vi "ADAM_scan_table.vi"() -> ()   [LabVIEW 2013]
uses:
  Anemometry/Anemometry Sub Vis/Controls/Serveds.ctl
  ADAM Client/Sub VIs/ADAM Controls/Module_type_ADAM.ctl
  ADAM Client/Sub VIs/ADAM Controls/Traverse_Level_State.ctl
  Anemometry/Anemometry Sub Vis/Controls/Post_Process.ctl
  ADAM Client/Sub VIs/ADAM Controls/Channel_State.ctl
  ADAM Client/Sub VIs/ADAM Controls/Ch_description_ADAM.ctl
  ADAM Client/Sub VIs/ADAM Controls/Function_ADAM.ctl
  ADAM Client/Sub VIs/ADAM Controls/Calib_type_ADAM.ctl
  ADAM Client/Sub VIs/ADAM Controls/Address.ctl
  ADAM_Global.vi
  Sub VI's/Channel_Description_Global.vi
  Anemometry/Anemometry Sub Vis/Globals/Meas_global.vi
  Sub VI's/Logged_Data_real_Global.vi
  Anemometry/Anemometry Sub Vis/Globals/Preference_global.vi
  Anemometry/Anemometry Sub Vis/Globals/Gas_management_global.vi
  Anemometry/Anemometry Sub Vis/Globals/Constants_global.vi
panel:
  in  "Reconfigure Gills":bool
  in  "Full Res Pathname":path
  in  "Log full Res Data":bool
  out "Duty No":u16 format="%.0b"
  in  "Save Current setup":bool=TRUE
  in  "Load setup from file":bool
  out "ADAM scan comments":string
  out "History length":i32=250
  in  "stop":bool
  out "Results":dbl[](array[numeric]) format="%.3f"
  out "Titles":string[](array[string])
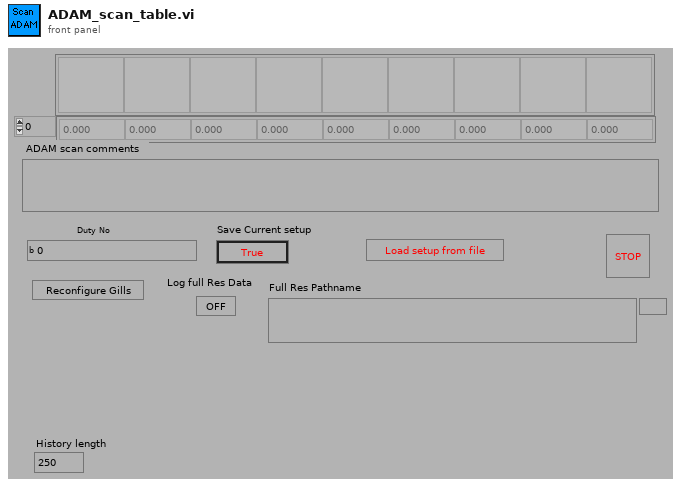
[diagram p1: front panel]
types:
  T1 = enum16{"Load ADAM setup from excel file", "Save ADAM setup to excel file"}
  T2 = typedef "Serveds.ctl" = enum16{"Read Global", "Load Global From File"}
  T3 = typedef "Module_type_ADAM.ctl" = string
  T4 = typedef "Traverse_Level_State.ctl" = enum16{"Running", "Complete"}
  T5 = typedef "Post_Process.ctl" = enum16{"Take New Data", "Post Process Raw Data File"}
  T6 = typedef "Channel_State.ctl" = enum16{"On", "Off", "Always On", "Always Off"}
  T7 = enum16{"Append to Global", "Read Global then Clear"}
  T8 = typedef "Ch_description_ADAM.ctl" = cluster{"Ch Name":string, "Type":T3, "Function":T9, "Ch State":T6, "Calibration type":T10, "A":dbl, "B":dbl, "C":dbl, "D":dbl, "Comments":string, "Address":T11, "String":string, "Duty":u16}
  T9 = typedef "Function_ADAM.ctl" = enum16{"Analogue Input", "Digital Input", "Event counter", "Event rate", "Analogue Output", "Digital Output", "Relay Output"}
  T10 = typedef "Calib_type_ADAM.ctl" = enum16{"Raw", "Bx + A", "Cx^2 + Bx + A", "Dx^3 + Cx^2 + Bx + A", "In Band", "Hi-Tec Q", "Hi-Tec M_dot", "Text"}
  T11 = typedef "Address.ctl" = cluster{"Main":i32, "Ch.":i32, "Sub":i32, "Port Name":string}
  T12 = typedef "Client_State_Cluster.ctl" = cluster{"Client Name":string, "Traverse level State":T4, "People to Email":string[], "Next Contact Time":dbl}
  T13 = typedef "ADAM_Comparitor.ctl" = cluster{"Ch to Monitor":string, "Channels to Kill":string, "Warn if Above":dbl, "Warn if Below":dbl, "Kill if Above":dbl, "Kill if Below":dbl, "Hysteresis Margin":dbl, "Averaging TIme (s)":dbl, "Warn Status":bool, "Kill Status":bool, "Extra Email addresses":string}
  T14 = typedef "Update_scan_value.ctl" = cluster{"Channel Name":string, "New Value":dbl}
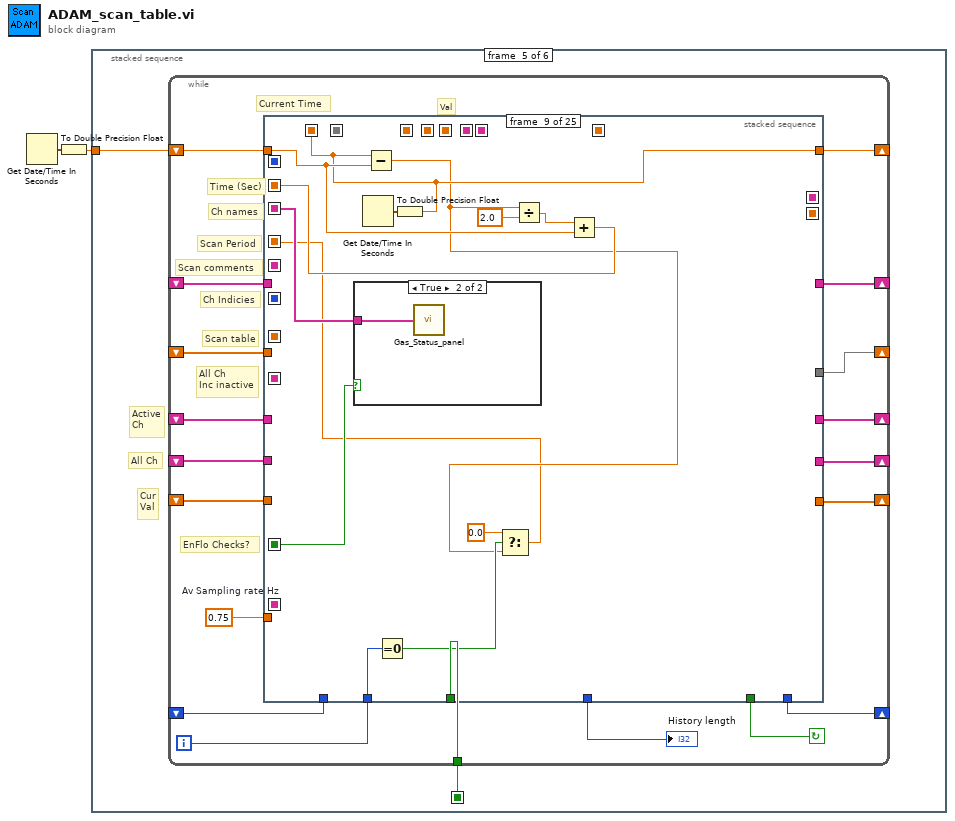
[diagram p0: block diagram]
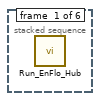
[diagram p2: hidden frame]
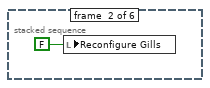
[diagram p3: hidden frame]
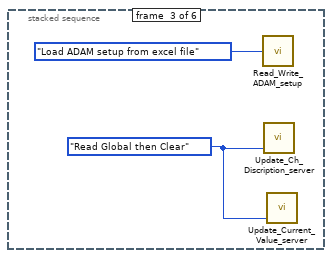
[diagram p4: hidden frame]
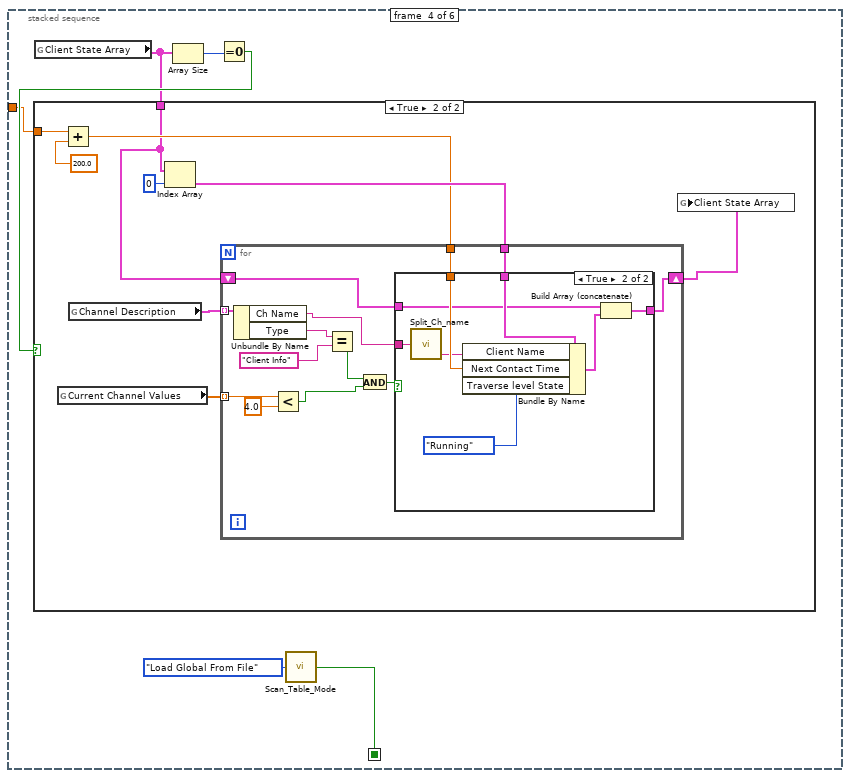
[diagram p5: hidden frame]
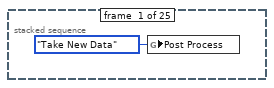
[diagram p8: hidden frame]
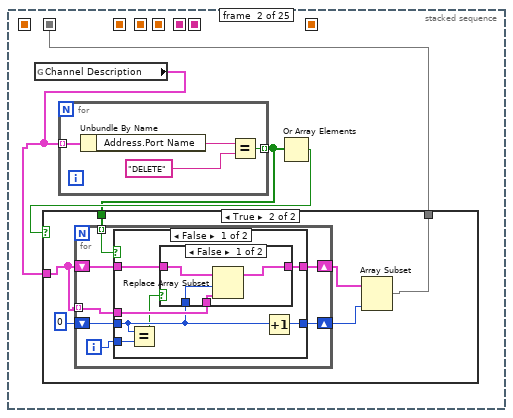
[diagram p9: hidden frame]
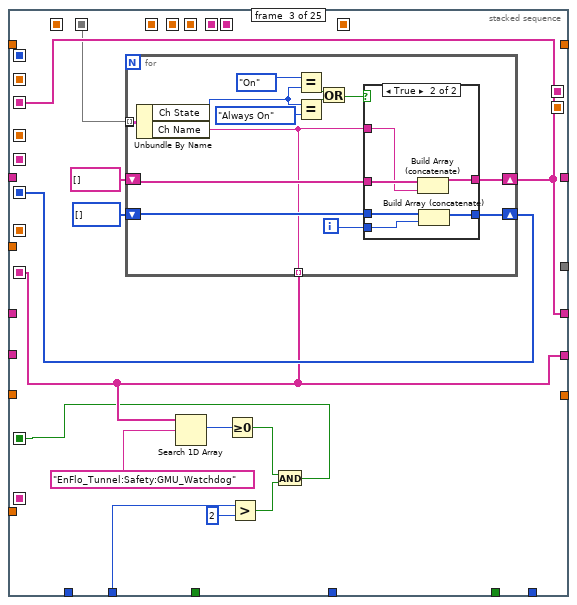
[diagram p13: hidden frame]
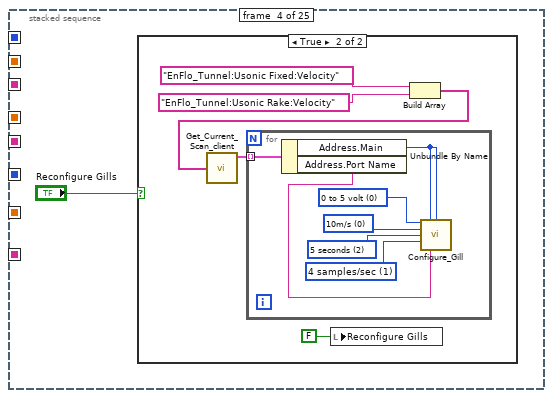
[diagram p15: hidden frame]
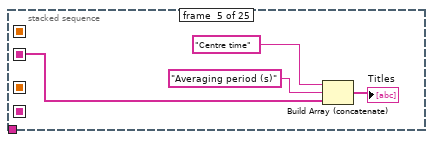
[diagram p17: hidden frame]
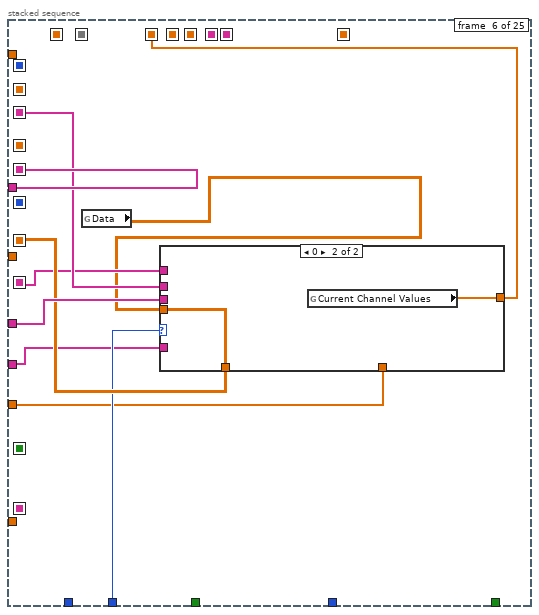
[diagram p18: hidden frame]
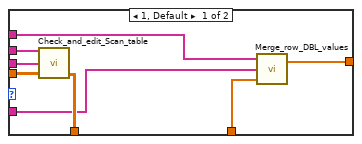
[diagram p19: hidden frame]
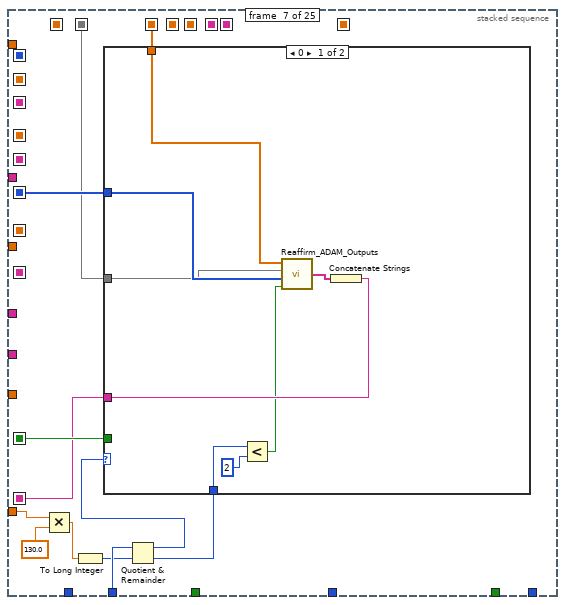
[diagram p20: hidden frame]
diagram:
  n1 = Get Date/Time In Seconds() -> (seconds since 1Jan1904=w2:timestamp)
  n2 = To Double Precision Float(number=w2) -> (double precision float=w1:dbl)
  n3 = stacked-sequence {
    seq-local: [_ _ _ w11 _ _] -> [_ _ _ _ w44 _]
    tunnel: w1 -> [_ _ _ w6 w43 _]
    frame #0 {
      n4 = call "Run_EnFlo_Hub.vi"() -> ()  [unwired: 8 out]
    }
    frame #1 {
      n5 = local write "Reconfigure Gills"(FALSE ("Reconfigure Gills")) -> ()
    }
    frame #2 {
      w4 = T7."Read Global then Clear" ("Mode")
      n6 = call "Read_Write_ADAM_setup.vi"("Mode"=T1."Load ADAM setup from excel file") -> ()  [unwired: 4 out]
      n7 = call "Update_Ch_Discription_server.vi"("Mode"=w4) -> ()  [unwired: 2 in, 1 out]
      n8 = call "Update_Current_Value_server.vi"("Mode"=w4) -> ()  [unwired: 2 in, 1 out]
    }
    frame #3 {
      n9 = global read "ADAM_Global.vi" "Client State Array"() -> (w7:T12[])
      n10 = Array Size(array=w7) -> (size(s)=w9:i32)
      n11 = Equal To 0?(x=w9) -> (x = 0?=w8:bool)
      n12 = case shown="True" w8 {
        tunnel: w7 -> [_ w13]
        tunnel: w6 -> [_ w16]
        frame False {
        }
        frame True {
          n13 = global read "ADAM_Global.vi" "Current Channel Values"() -> (w20:dbl[])
          n14 = Add(x=w16, y=200.0) -> (x+y=w14:dbl)
          n15 = global read "Channel_Description_Global.vi" "Channel Description"() -> (w19:T8[])
          n16 = Index Array(array=w13, index=0) -> (element=w17:T12)
          n17 = for {
            tunnel: w19 -> [w33] mode=indexing
            tunnel: w20 -> [w25] mode=indexing
            tunnel: w17 -> [w26]
            tunnel: w14 -> [w24]
            shift-right: [w23] -> w12
            shift-left: w13 -> [w22]
            n18 = Unbundle By Name(w33) -> ("Ch Name"=w21:string, "Type"=w30:T3)
            n19 = Less?(x=w25, y=4.0) -> (x < y?=w28:bool)
            n20 = Equal?(x=w30, y=T3 "Client Info" ("Type")) -> (x = y?=w29:bool)
            n21 = And(x=w29, y=w28) -> (x .and. y?=w27:bool)
            n22 = case shown="True" w27 {
              tunnel: w26 -> [_ w42]
              tunnel: w24 -> [_ w41]
              tunnel: [w34 w39] -> w23
              tunnel: w22 -> [w34 w38]
              tunnel: w21 -> [_ w36]
              frame False {
              }
              frame True {
                n23 = call "Split_Ch_name.vi"("Ch name"=w36) -> ("Low level"=w35:string)  [unwired: 2 out]
                n24 = Bundle By Name(cluster=w42, "Client Name"=w35, "Next Contact Time"=w41, "Traverse level State"=Traverse_Level_State."Running") -> (w37:T12)
                n25 = Build Array (concatenate)(w38, w37) -> (w39:T12[])
              }
            }
          }
          n26 = global write "ADAM_Global.vi" "Client State Array"(w12) -> ()
        }
      }
      n27 = call "Scan_Table_Mode.vi"("Mode"=Serveds."Load Global From File") -> ("Simulate Mode ?"=w11:bool)
    }
    frame #4 {
      # "Active\nCh"
      # "Cur\nVal"
      # "All Ch"
      n28 = while {
        shift-left: _ -> [w47]
        shift-right: [w46] -> _
        shift-left: _ -> [w48]
        shift-right: [w49] -> _
        shift-left: _ -> [w50]
        shift-right: [w51] -> _
        tunnel: w44 -> [w52]
        shift-left: _ -> [w55]
        shift-right: [w54] -> _
        shift-left: _ -> [w57]
        shift-right: [w58] -> _
        shift-left: _ -> [w59]
        shift-right: [w60] -> _
        shift-left: w43 -> [w61]
        shift-right: [w62] -> _
        i -> [w56]
        stop <- w63 continue-if-true
        w45 = 0.75  # Av Sampling rate Hz
        # "Current Time"
        # "EnFlo Checks?"
        # "Val"
        # "All Ch\nInc inactive"
        # "Scan comments"
        # "Scan table"
        # "Time (Sec)"
        # "Ch Indicies"
        # "Ch names"
        # "Scan Period"
        n29 = stacked-sequence {
          seq-local: [_ _ _ _ _ _ _ _ _ _ _ _ _ _ _ w313 _ _ _ _ _ _ _ _ _] -> [_ _ _ _ _ _ _ _ _ _ _ _ _ _ _ _ _ w364 w369 _ _ _ _ w447 _]
          seq-local: [_ _ _ _ _ _ _ _ w208 _ _ _ _ _ _ _ _ _ _ _ _ _ _ _ _] -> [_ _ _ _ _ _ _ _ _ _ _ _ _ _ _ _ _ _ w376 _ _ _ _ _ _]
          seq-local: [_ _ _ _ _ w158 _ _ _ _ _ _ _ _ _ _ _ _ _ _ _ _ _ _ _] -> [_ _ _ _ _ _ _ w196 _ _ _ _ _ _ _ _ _ _ w374 _ _ _ _ _ _]
          seq-local: [_ _ _ _ _ _ _ _ w200 _ _ _ _ _ _ _ _ _ _ _ _ _ _ _ _] -> [_ _ _ _ _ _ _ _ _ _ w234 _ _ _ _ _ _ _ w375 _ _ _ _ _ _]
          seq-local: [_ _ _ _ _ w161 _ _ _ _ _ _ _ _ _ _ _ _ _ _ _ _ _ _ _] -> [_ _ _ _ _ _ _ w198 _ _ _ _ _ _ _ _ _ _ _ _ w414 _ _ _ _]
          seq-local: [_ _ _ _ _ _ _ _ _ _ w232 _ _ _ _ _ _ _ _ _ _ _ _ _ _] -> [_ _ _ _ _ _ _ _ _ _ _ w251 _ _ _ _ _ _ _ _ _ _ _ _ _]
          seq-local: [_ _ w112 _ _ _ _ _ _ _ _ _ _ _ _ _ _ _ _ _ _ _ _ _ _] -> [_ _ _ _ w150 w160 _ w199 w212 _ _ _ _ _ _ _ _ _ w372 w377 _ _ _ _ _]
          seq-local: [_ _ w111 _ _ _ _ _ _ _ _ _ _ _ _ _ _ _ _ _ _ _ _ _ _] -> [_ _ _ _ _ _ w176 w194 _ _ w233 _ _ _ _ _ _ _ _ _ _ _ _ _ _]
          seq-local: [_ _ _ _ _ w154 _ _ _ _ _ _ _ _ _ _ _ _ _ _ _ _ _ _ _] -> [_ _ _ _ _ _ w174 w195 _ _ w230 _ _ _ _ _ _ _ _ _ _ _ _ _ _]
          seq-local: [_ _ _ _ _ _ _ _ _ _ w228 _ _ _ _ _ _ _ _ _ _ _ _ _ _] -> [_ _ _ _ _ _ _ _ _ _ _ w256 w285 _ _ w311 _ _ _ _ _ _ _ _ _]
          seq-local: [_ _ w107 _ _ _ _ _ _ _ _ _ _ _ _ _ _ _ _ _ _ _ _ _ _] -> [_ _ _ _ _ w156 _ w197 _ _ w229 w255 w284 _ _ w312 w337 w356 w371 _ _ _ w424 _ _]
          seq-local: [_ _ _ _ _ _ _ _ _ w214 _ _ _ _ _ _ _ _ _ _ _ _ _ _ _] -> [_ _ _ _ _ _ _ _ _ _ w227 _ _ _ _ _ _ _ _ _ _ _ _ _ _]
          seq-local: [_ w65 _ _ _ _ _ _ _ _ _ _ _ _ _ _ _ _ _ _ _ _ _ _ _] -> [_ _ w109 _ _ _ w175 w193 _ _ w226 _ _ _ _ _ _ _ _ _ _ _ _ _ _]
          seq-local: [_ _ _ _ _ _ _ _ w207 _ _ _ _ _ _ _ _ _ _ _ _ _ _ _ _] -> [_ _ _ _ _ _ _ _ _ _ _ w252 _ _ _ _ _ _ _ w379 _ _ _ _ _]
          seq-local: [_ _ _ _ _ _ _ _ _ _ _ _ _ _ _ _ _ _ w368 _ _ _ _ _ _] -> [_ _ _ _ _ _ _ _ _ _ _ _ _ _ _ _ _ _ _ w378 _ _ _ _ _]
          seq-local: [_ _ w101 _ _ _ _ _ _ _ _ _ _ _ _ _ _ _ _ _ _ _ _ _ _] -> [_ _ _ _ _ _ w183 _ w205 _ _ w254 w283 w297 w306 _ _ _ _ _ _ _ _ _ w451]
          seq-local: [_ _ _ _ _ _ _ _ _ _ _ _ _ _ _ w310 _ _ _ _ _ _ _ _ _] -> [_ _ _ _ _ _ _ _ _ _ _ _ _ _ _ _ w338 _ _ _ _ _ _ _ _]
          seq-local: [_ _ _ _ _ _ w173 _ _ _ _ _ _ _ _ _ _ _ _ _ _ _ _ _ _] -> [_ _ _ _ _ _ _ _ _ _ w225 _ _ _ _ _ _ _ _ _ _ _ _ _ _]
          seq-local: [_ _ _ _ _ _ _ _ _ _ _ _ _ _ _ w309 _ _ _ _ _ _ _ _ _] -> [_ _ _ _ _ _ _ _ _ _ _ _ _ _ _ _ w336 _ _ _ _ _ _ _ _]
          seq-local: [_ _ _ _ _ _ _ _ _ _ _ w250 _ _ _ _ _ _ _ _ _ _ _ _ _] -> [_ _ _ _ _ _ _ _ _ _ _ _ _ _ _ _ _ _ _ _ w402 _ _ _ _]
          tunnel: [_ _ _ _ _ _ _ _ _ _ _ _ _ _ _ _ _ _ _ _ _ w422 _ _ _] -> w63
          tunnel: [_ _ _ _ _ _ _ _ w207 _ _ _ _ _ _ _ _ _ _ _ _ _ _ _ _] -> w62
          tunnel: w61 -> [_ _ _ _ _ _ _ _ w209 _ _ _ _ _ _ _ _ _ _ _ _ _ _ _ _]
          tunnel: [_ _ _ _ _ _ _ _ _ _ _ _ _ _ _ _ _ _ _ _ w412 _ _ _ _] -> w60
          tunnel: w59 -> [_ _ _ _ _ w161 _ _ _ _ _ _ _ _ _ _ _ _ _ _ _ _ _ _ _]
          tunnel: [_ _ w112 _ _ _ _ _ _ _ _ _ _ _ _ _ _ _ _ _ _ _ _ _ _] -> w58
          tunnel: w57 -> [_ _ _ _ _ w159 _ _ _ _ _ _ _ _ _ _ w339 _ _ _ _ _ _ _ _]
          tunnel: w56 -> [_ _ w105 _ _ w157 w179 _ w204 _ _ w253 w279 w293 w302 _ _ _ _ _ _ w420 _ _ w452]
          tunnel: w55 -> [_ _ _ _ _ _ _ _ _ _ _ _ _ _ _ _ _ w362 _ _ _ _ _ _ _]
          tunnel: [_ _ _ _ _ _ _ _ _ _ _ _ _ _ _ _ _ w358 _ _ _ _ _ _ _] -> w54
          tunnel: [_ _ _ _ _ _ _ _ _ _ _ _ _ _ _ _ _ _ w373 _ _ _ _ _ _] -> w53
          tunnel: w52 -> [_ _ _ _ _ _ _ _ _ _ w231 _ _ _ _ _ _ _ _ _ _ _ _ _ _]
          tunnel: [_ _ w107 _ _ _ _ _ _ _ _ _ _ _ _ _ _ _ _ _ _ _ _ _ _] -> w51
          tunnel: w50 -> [_ _ _ _ _ w155 _ _ _ _ _ _ _ _ _ _ _ _ _ _ _ _ _ _ _]
          tunnel: [_ _ _ _ _ _ _ _ _ _ _ _ _ _ _ _ _ _ _ _ _ _ _ w447 _] -> w49
          tunnel: w48 -> [_ _ _ _ _ w153 _ _ _ _ _ _ _ _ _ _ _ _ _ _ _ _ _ _ _]
          tunnel: w47 -> [_ _ _ _ _ _ _ _ _ w215 _ _ _ _ _ _ _ _ _ _ _ _ _ _ _]
          tunnel: [_ _ _ _ _ _ _ _ _ w216 _ _ _ _ _ _ _ _ _ _ _ _ _ _ _] -> w46
          tunnel: w45 -> [_ _ _ _ _ _ w182 _ _ _ _ _ w282 w296 w305 _ _ _ _ _ _ _ _ _ _]
          frame #0 {
            n30 = global write "Meas_global.vi" "Post Process"(Post_Process."Take New Data" ("Post Process")) -> ()
          }
          frame #1 {
            n31 = global read "Channel_Description_Global.vi" "Channel Description"() -> (w67:T8[])
            n32 = for {
              tunnel: w67 -> [w100] mode=indexing
              tunnel: [w97] -> w66 mode=indexing
              n33 = Unbundle By Name(w100) -> ("Address.Port Name"=w99:string)
              n34 = Equal?(x=w99, y="DELETE") -> (x = y?=w97:bool)
            }
            n35 = Or Array Elements(Boolean array=w66) -> (logical OR=w68:bool)
            n36 = case shown="True" w68 {
              tunnel: w67 -> [w69 w73]
              tunnel: w66 -> [_ w75]
              tunnel: [w69 w70] -> w65
              frame False {
              }
              frame True {
                n37 = for {
                  shift-right: [w82] -> w72
                  shift-left: w73 -> [w81]
                  tunnel: w75 -> [w77] mode=indexing
                  shift-right: [w80] -> w71
                  shift-left: 0 -> [w78]
                  tunnel: w73 -> [w79] mode=indexing
                  i -> [w76]
                  n38 = case shown="False" w77 {
                    tunnel: [w88 w96] -> w82
                    tunnel: w81 -> [w89 w96]
                    tunnel: [w86 w95] -> w80
                    tunnel: w78 -> [w85 w95]
                    tunnel: w79 -> [w87 _]
                    tunnel: w76 -> [w84 _]
                    frame False {
                      n39 = Equal?(x=w85, y=w84) -> (x = y?=w83:bool)
                      n40 = case shown="False" w83 {
                        tunnel: w89 -> [w93 w94]
                        tunnel: [w92 w94] -> w88
                        tunnel: w87 -> [w91 _]
                        tunnel: w85 -> [w90 _]
                        frame False {
                          n41 = Replace Array Subset(array=w93, new element=w91, index=w90) -> (w92:T8[])
                        }
                        frame True {
                        }
                      }
                      n42 = Increment(x=w85) -> (x+1=w86:i32)
                    }
                    frame True {
                    }
                  }
                }
                n43 = Array Subset(array=w72, length=w71) -> (w70:T8[])  [unwired: 1 in]
              }
            }
          }
          frame #2 {
            n44 = for {
              tunnel: [w126] -> _ mode=indexing
              shift-right: [w125] -> w112
              shift-left: string[] [] -> [w116]
              shift-right: [w122] -> w111
              shift-left: i32[] [] -> [w124]
              tunnel: [w114] -> w107 mode=indexing
              tunnel: w109 -> [w126] mode=indexing
              i -> [w123]
              n45 = Unbundle By Name(w126) -> ("Ch State"=w117:T6, "Ch Name"=w114:string)
              n46 = Equal?(x=Channel_State."On" ("Channel State"), y=w117) -> (x = y?=w119:bool)
              n47 = Equal?(x=w117, y=Channel_State."Always On" ("Channel State")) -> (x = y?=w118:bool)
              n48 = Or(x=w119, y=w118) -> (x .or. y?=w115:bool)
              n49 = case shown="True" w115 {
                tunnel: w116 -> [w127 w134]
                tunnel: w114 -> [_ w133]
                tunnel: [w127 w132] -> w125
                tunnel: w124 -> [w128 w131]
                tunnel: w123 -> [_ w130]
                tunnel: [w128 w129] -> w122
                frame False {
                }
                frame True {
                  n50 = Build Array (concatenate)(w134, w133) -> (w132:string[])
                  n51 = Build Array (concatenate)(w131, w130) -> (w129:i32[])
                }
              }
            }
            n52 = Search 1D Array(1D array=w107, element="EnFlo_Tunnel:Safety:GMU_Watchdog") -> (index of element=w106:i32)  [unwired: 1 out]
            n53 = Greater Or Equal To 0?(x=w106) -> (x >= 0?=w102:bool)
            n54 = Greater?(x=w105, y=2) -> (0:w103:bool)
            n55 = And(x=w102, y=w103) -> (x .and. y?=w101:bool)
          }
          frame #3 {
            n56 = case shown="True" "Reconfigure Gills" {
              frame False {
              }
              frame True {
                n57 = local write "Reconfigure Gills"(FALSE ("Reconfigure Gills")) -> ()
                n58 = Build Array("EnFlo_Tunnel:Usonic Fixed:Velocity", "EnFlo_Tunnel:Usonic Rake:Velocity") -> (w138:string[])
                n59 = call "Get_Current_Scan_client.vi"("ADAM Ch Names"=w138) -> ("Ch Description Array"=w137:T8[])  [unwired: 3 out]
                n60 = for {
                  tunnel: w137 -> [w143] mode=indexing
                  w147 = u16 1 items=["1 sample/sec", "4 samples/sec"] ("Samples/sec")
                  w146 = u16 2 items=["OFF", "3 seconds", "5 seconds", "10 seconds"] ("Averaging Time")
                  w145 = u16 0 items=["10m/s", "20m/s", "30m/s", "40m/s", "50m/s", "60m/s", "70m/s"] ("Analogue O/P Scale")
                  w144 = u16 0 items=["0 to 5 volt", "+/-2.5 Volt", "4-20mA"] ("Analogue O/P Config")
                  n61 = Unbundle By Name(w143) -> ("Address.Main"=w142:i32, "Address.Port Name"=w141:string)
                  n62 = call "Configure_Gill.vi"("Analogue O/P Config"=w144, "ORIGINAL Address"=w142, "NEW Address"=w142, "Analogue O/P Scale"=w145, "Averaging Time"=w146, "Samples/sec"=w147, "Port Name"=w141) -> ()  [unwired: 9 out]
                }
              }
            }
          }
          frame #4 {
            n63 = Build Array (concatenate)("Centre time", "Averaging period (s)", w150) -> (→"Titles":string[])
          }
          frame #5 {
            n64 = global read "Logged_Data_real_Global.vi" "Data"() -> (w152:dbl[][])
            n65 = case shown="0" w157 {
              tunnel: w152 -> [w169 w171]
              tunnel: w160 -> [w166 _]
              tunnel: w159 -> [w168 _]
              tunnel: [w167 w171] -> w158
              tunnel: w156 -> [w165 _]
              tunnel: w155 -> [w164 _]
              tunnel: [w163 w170] -> w154
              tunnel: w153 -> [w162 _]
              frame 1, Default {
                n66 = call "Check_and_edit_Scan_table.vi"("2D array input"=w169, "Original Channels"=w168, "Present Channels"=w166) -> ("2D array output"=w167:dbl[][])  [unwired: 2 out]
                n67 = call "Merge_row_DBL_values.vi"("Present Row values"=w162, "Present Channels"=w164, "Desired Channels"=w165) -> ("Desired Row values"=w163:dbl[])  [unwired: 1 out]
              }
              frame 0 {
                n68 = global read "ADAM_Global.vi" "Current Channel Values"() -> (w170:dbl[])
              }
            }
          }
          frame #6 {
            n69 = Multiply(x=w182, y=130.0) -> (x*y=w180:dbl)
            n70 = To Long Integer(number=w180) -> (32bit integer=w178:i32)
            n71 = Quotient & Remainder(x=w179, y=w178) -> (x-y*floor(x/y)=w177:i32, floor(x/y)=w172:i32)
            n72 = case shown="0" w177 {
              tunnel: w183 -> [_ _]
              tunnel: w176 -> [w190 _]
              tunnel: w175 -> [w189 _]
              tunnel: w174 -> [w188 _]
              tunnel: [w187 ""] -> w173
              tunnel: w172 -> [w185 _]
              frame 0 {
                n73 = Less?(x=w185, y=2) -> (x < y?=w186:bool)
                n74 = call "Reaffirm_ADAM_Outputs.vi"("Reset Zeros as well"=w186, "Active Ch Indicies"=w190, "Channel Description"=w189, "Current Channel Values"=w188) -> ("Scan Comments"=w191:string[])  [unwired: 2 in]
                n75 = Concatenate Strings(w191) -> (w187:string)
              }
              frame 1, Default {
              }
            }
          }
          frame #7 {
            n76 = global write "ADAM_Global.vi" "Active Ch names"(w199) -> ()
            n77 = global write "ADAM_Global.vi" "Scan comments"(w198) -> ()
            n78 = global write "Channel_Description_Global.vi" "Channel Description"(w193) -> ()
            n79 = global write "ADAM_Global.vi" "Active Ch Indicies"(w194) -> ()
            n80 = global write "ADAM_Global.vi" "All Ch names"(w197) -> ()
            n81 = global write "Logged_Data_real_Global.vi" "Data"(w196) -> ()
            n82 = global write "ADAM_Global.vi" "Current Channel Values"(w195) -> ()
          }
          frame #8 {
            n83 = case shown="True" w205 {
              tunnel: w212 -> [_ w213]
              frame False {
              }
              frame True {
                n84 = call "Gas_Status_panel.vi"("Ch names"=w213) -> ()  [unwired: 15 out]
              }
            }
            n85 = Get Date/Time In Seconds() -> (seconds since 1Jan1904=w206:timestamp)
            n86 = Equal To 0?(x=w204) -> (x = 0?=w203:bool)
            n87 = To Double Precision Float(number=w206) -> (double precision float=w207:dbl)
            n88 = Subtract(x=w207, y=w209) -> (x-y=w202:dbl)
            n89 = Select(t=0.0, s=w203, f=w202) -> (s? t:f=w200:dbl)
            n90 = Divide(x=w202, y=2.0) -> (x/y=w210:dbl)
            n91 = Add(x=w210, y=w209) -> (x+y=w208:dbl)
          }
          frame #9 {
            n92 = Equal To 0?(x=w215) -> (x = 0?=w219:bool)
            n93 = Equal?(x=u16 32768, y=w215) -> (x = y?=w218:bool)
            n94 = Select(t=u16 1, s=w219, f=w215) -> (s? t:f=w214:u16)
            "Duty No" <- w214
            n95 = case shown="False" w218 {
              tunnel: [w221 u16 0] -> w216
              tunnel: w214 -> [w223 _]
              frame False {
                n96 = Multiply(x=u16 2, y=w223) -> (x*y=w221:u16)
              }
              frame True {
              }
            }
          }
          frame #10 {
            n97 = for {
              tunnel: w226 -> [w241]
              tunnel: w234 -> [w249]
              shift-right: [w247] -> w228
              shift-left: w230 -> [w245]
              tunnel: w229 -> [w246]
              shift-right: [w242] -> w232
              shift-left: w225 -> [w244]
              tunnel: w233 -> [w236] mode=indexing
              tunnel: w230 -> [w238]
              tunnel: w231 -> [w239]
              tunnel: w227 -> [w235]
              n98 = Index Array(array=w238, index=w236) -> (element=w237:dbl)
              n99 = Index Array(array=w241, index=w236) -> (element=w240:T8)
              n100 = call "Adam_Ch_Input_Output.vi"("Simulate"=w239, "Duty No"=w235, "Previuos Scan Value"=w237, "Ch values"=w245, "Scan Period"=w249, "Ch Discription"=w240, "Ch names"=w246) -> ("Scan comment"=w243:string, "Calibrated units"=w248:dbl)  [unwired: 1 in, 2 out]
              n101 = Concatenate Strings(w244, w243) -> (w242:string)
              n102 = Replace Array Subset(array=w245, new element=w248, index=w236) -> (w247:dbl[])
            }
          }
          frame #11 {
            n103 = case shown="True" w254 {
              tunnel: w256 -> [_ w263]
              tunnel: w255 -> [_ w262]
              tunnel: w253 -> [_ w261]
              tunnel: w252 -> [_ w271]
              tunnel: w251 -> [w258 w260]
              tunnel: [w258 w268] -> w250
              frame False {
              }
              frame True {
                n104 = global read "ADAM_Global.vi" "Comparitor Array"() -> (w267:T13[])
                n105 = for {
                  tunnel: w267 -> [w276] mode=indexing
                  tunnel: [w275] -> w266 mode=indexing
                  tunnel: w263 -> [w274]
                  tunnel: w262 -> [w273]
                  tunnel: [w272] -> w265 mode=indexing
                  n106 = call "ADAM_Comparitor.vi"("Comparator Info"=w276, "Ch names"=w273, "Present scan array"=w274) -> ("Comparator Info Out"=w275:T13, "Scan comment"=w272:string)  [unwired: 1 in]
                }
                n107 = call "LDA1_Safety.vi"("Adam Loop Count"=w261, "Ch Names"=w262, "Values"=w263) -> ("Scan comment"=w259:string)
                n108 = call "LDA2_Safety.vi"("Adam Loop Count"=w261, "Ch Names"=w262, "Values"=w263) -> ("Scan comment"=w264:string)
                n109 = call "Safety_Check.vi"("Adam Loop Count"=w261, "Ch Names"=w262, "Values"=w263) -> ("Scan comment"=w270:string)
                n110 = call "Check_Aero_Tunnel_on_Server.vi"("Values"=w263, "Ch Names"=w262, "Current Time"=w271, "Adam Loop Count"=w261) -> ("Scan comment"=w269:string)  [unwired: 2 in]
                n111 = global write "ADAM_Global.vi" "Comparitor Array"(w266) -> ()
                n112 = Concatenate Strings(w260, w259, w264, w270, w269, w265) -> (w268:string)
              }
            }
            n113 = property on="Results" class="Arr (strict)"() -> ("Index Values"=w257:u32[])  [unwired: 2 in, 2 out]
            n114 = property on="Titles" class="Arr (strict)"("Index Values"=w257) -> ()  [unwired: 2 in, 2 out]
          }
          frame #12 {
            n115 = Multiply(x=w282, y=60.0) -> (x*y=w280:dbl)
            n116 = To Long Integer(number=w280) -> (32bit integer=w278:i32)
            n117 = Quotient & Remainder(x=w279, y=w278) -> (x-y*floor(x/y)=w277:i32)  [unwired: 1 out]
            n118 = case shown="0" w277 {
              tunnel: w285 -> [w288 _]
              tunnel: w284 -> [w287 _]
              tunnel: w283 -> [w286 _]
              frame 0 {
                n119 = case shown="True" w286 {
                  tunnel: w288 -> [_ w290]
                  tunnel: w287 -> [_ w289]
                  frame False {
                  }
                  frame True {
                    n120 = call "Do_Every_minute.vi"("Ch Names"=w289, "Values"=w290) -> ()  [unwired: 1 out]
                  }
                }
              }
              frame 1, Default {
              }
            }
          }
          frame #13 {
            n121 = Multiply(x=w296, y=350.0) -> (x*y=w294:dbl)
            n122 = To Long Integer(number=w294) -> (32bit integer=w292:i32)
            n123 = Quotient & Remainder(x=w293, y=w292) -> (x-y*floor(x/y)=w291:i32)  [unwired: 1 out]
            n124 = case shown="0" w291 {
              tunnel: w297 -> [w298 _]
              frame 0 {
                n125 = case shown="True" w298 {
                  frame False {
                  }
                  frame True {
                    w299 = TRUE  # Set Watchdogs
                    n126 = call "Set_Adam_Watchdogs.vi"("Set Watchdogs"=w299) -> ()  [unwired: 1 out]
                  }
                }
              }
              frame 1, Default {
              }
            }
          }
          frame #14 {
            n127 = Multiply(x=w305, y=55.0) -> (x*y=w303:dbl)
            n128 = To Long Integer(number=w303) -> (32bit integer=w301:i32)
            n129 = Quotient & Remainder(x=w302, y=w301) -> (x-y*floor(x/y)=w300:i32)  [unwired: 1 out]
            n130 = case shown="0" w300 {
              tunnel: w306 -> [_ _]
              frame 0 {
                n131 = case shown="True" "Save Current setup" {
                  frame False {
                  }
                  frame True {
                    n132 = call "Read_Write_ADAM_setup.vi"("Mode"=T1."Save ADAM setup to excel file") -> ()  [unwired: 4 out]
                  }
                }
              }
              frame 1, Default {
              }
            }
          }
          frame #15 {
            n133 = call "Update_Current_Value_server.vi"("Mode"=T7."Read Global then Clear") -> ("Update array out"=w315:T14[])  [unwired: 2 in]
            n134 = for {
              tunnel: w312 -> [w323]
              tunnel: w315 -> [w318] mode=indexing
              shift-right: [w321] -> w313
              shift-left: w311 -> [w322]
              tunnel: [w317] -> w310 mode=indexing
              tunnel: [w316] -> w309 mode=indexing
              n135 = Unbundle By Name(w318) -> ("Channel Name"=w317:string, "New Value"=w316:dbl)
              n136 = Search 1D Array(1D array=w323, element=w317) -> (index of element=w320:i32)  [unwired: 1 out]
              n137 = Less Than 0?(x=w320) -> (x < 0?=w319:bool)
              n138 = case shown="True" w319 {
                tunnel: w317 -> [_ w324]
                tunnel: w318 -> [_ w329]
                frame False {
                }
                frame True {
                  n139 = global read "ADAM_Global.vi" "Update Current Value"() -> (w328:T14[])
                  n140 = call "Check_Ch_Name_colons.vi"("No of Colons"=2, "Ch Name in"=w324) -> ("Ch Name out"=w325:string)
                  n141 = Bundle By Name(cluster=T8 {"Ch Name"="", "Type"="Hold Value", "Function"=enum."Analogue Input", "Ch State"=enum."On", "Calibration type"=enum."Raw", "A"=0.0, "B"=0.0, "C"=0.0, "D"=0.0, "Comments"="", "Address"={"Main"=0, "Ch."=0, "Sub"=0, "Port Name"=""}, "String"="", "Duty"=0} ("Ch Description"), "Ch Name"=w325, "Type"=T3 "Hold Value") -> (w333:T8)
                  n142 = Build Array (concatenate)(w328, w329) -> (w327:T14[])
                  n143 = global write "ADAM_Global.vi" "Update Current Value"(w327) -> ()
                  n144 = global read "Preference_global.vi" "Rig Setup"() -> (w331:string)
                  n145 = Build Array(w333) -> (w332:T8[])
                  n146 = call "Update_Ch_Discription_server.vi"("Mode"=T7."Append to Global", "Client HD name"=w331, "Channels to update In"=w332) -> ()  [unwired: 1 out]
                }
              }
              n147 = Replace Array Subset(array=w322, new element=w316, index=w320) -> (w321:dbl[])
            }
          }
          frame #16 {
            n148 = for {
              tunnel: w339 -> [w347]
              tunnel: w338 -> [w345] mode=indexing
              tunnel: w337 -> [w346]
              tunnel: w336 -> [w343] mode=indexing
              n149 = Search 1D Array(1D array=w347, element=w345) -> (index of element=w344:i32)  [unwired: 1 out]
              n150 = Less Than 0?(x=w344) -> (x < 0?=w342:bool)
              n151 = Not Equal To 0?(x=w343) -> (x != 0?=w341:bool)
              n152 = And(x=w341, y=w342) -> (x .and. y?=w340:bool)
              n153 = case shown="True" w340 {
                tunnel: w346 -> [_ w355]
                tunnel: w345 -> [_ w354]
                frame False {
                }
                frame True {
                  n154 = Search 1D Array(1D array=w355, element=w354) -> (index of element=w349:i32)  [unwired: 1 out]
                  n155 = global read "Channel_Description_Global.vi" "Channel Description"() -> (w350:T8[])
                  n156 = Index Array(array=w350, index=w349) -> (element=w353:T8)
                  n157 = Bundle By Name(cluster=w353, "Ch State"=Channel_State."On") -> (w351:T8)
                  n158 = Replace Array Subset(array=w350, new element=w351, index=w349) -> (w348:T8[])
                  n159 = global write "Channel_Description_Global.vi" "Channel Description"(w348) -> ()
                }
              }
            }
          }
          frame #17 {
            n160 = Search 1D Array(1D array=w356, element="GMU:Source:Release Temp") -> (index of element=w363:i32)  [unwired: 1 out]
            n161 = Index Array(array=w364, index=w363) -> (element=w361:dbl)
            n162 = Build Array (concatenate)(w361, w362) -> (w360:dbl[])
            n163 = Array Subset(array=w360, length=10 ("Array Length")) -> (w358:dbl[])  [unwired: 1 in]
            n164 = call "Mean_fr_NaN_data.vi"("Data"=w358) -> ("Mean value"=w357:dbl)  [unwired: 1 out]
            n165 = global write "Gas_management_global.vi" "Release temp (deg C)"(w357) -> ()
          }
          frame #18 {
            w366 = 500000  # Table size
            n166 = call "Merge_row_DBL_values.vi"("Present Row values"=w369, "Present Channels"=w371, "Desired Channels"=w372) -> ("Desired Row values"=w370:dbl[])  [unwired: 1 out]
            n167 = Build Array (concatenate)(w376, w375, w370) -> (w368:dbl[])
            "Results" <- w368
            n168 = call "Manipulate_Table.vi"("Table size"=w366, "Latest Row"=w368, "Table Input"=w374) -> ("History length"=w373:i32, "Table Output"=w367:dbl[][])  [unwired: 1 out]
            n169 = global write "Logged_Data_real_Global.vi" "Data"(w367) -> ()
          }
          frame #19 {
            n170 = case shown="True" "Log full Res Data" {
              tunnel: w379 -> [_ w392]
              tunnel: w378 -> [_ w391]
              tunnel: w377 -> [_ w390]
              frame False {
              }
              frame True {
                n171 = Build Array (concatenate)(w392, w391) -> (w389:dbl[])
                n172 = Number To Fractional String(number=w389) -> (F-format string=w387:string[])  [unwired: 3 out]
                n173 = call "Does_file_exist_(simple).vi"("Pathname"="Full Res Pathname") -> ("exists?"=w386:bool)
                n174 = Build Array (concatenate)("Current time", "Centre Time", "Averaging period (s)", w390) -> (w388:string[])
                n175 = case shown="False" w386 {
                  tunnel: w388 -> [w398 _]
                  tunnel: w387 -> [w397 w399]
                  tunnel: [w394 w400] -> w382
                  frame False {
                    n176 = Build Array(w398, w397) -> (w395:string[][])
                    n177 = Array To Spreadsheet String(array=w395, 3:"%s" ("format string")) -> (spreadsheet string=w394:string)  [unwired: 1 out]
                  }
                  frame True {
                    n178 = Array To Spreadsheet String(array=w399, 3:"%s" ("format string")) -> (spreadsheet string=w400:string)  [unwired: 1 out]
                  }
                }
                n179 = call "Write_File_Simple.vi"("append to file? (new file:F)"=TRUE, "character string"=w382, "file path"="Full Res Pathname") -> ()  [unwired: 2 out]
              }
            }
          }
          frame #20 {
            w410 = 150 ("length")
            w411 = 50  # History length
            n180 = String Subset(string=w402, length (rest)=w410) -> (substring=w404:string)  [unwired: 1 out]
            n181 = String Length(string=w404) -> (length=w409:i32)
            n182 = Equal?(x=w410, y=w409) -> (x = y?=w408:bool)
            n183 = Select(t=" Clipped ", s=w408, f="") -> (s? t:f=w405:string)
            n184 = Concatenate Strings(w405, w404) -> (w403:string)
            n185 = Build Array (concatenate)(w414, w403) -> (w413:string[])
            n186 = Array Size(array=w413) -> (size(s)=w416:i32)
            n187 = Subtract(x=w416, y=w411) -> (x-y=w415:i32)
            n188 = Array Subset(array=w413, index=w415) -> (w412:string[])  [unwired: 1 in]
            "ADAM scan comments" <- w402
          }
          frame #21 {
            n189 = Format Into String(format string="%s %d %s" ("Format String"), "\nScan No " ("Header message"), w420, "\r\n") -> (resulting string=w419:string)  [unwired: 2 in, 1 out]
            n190 = call "Write_out_serial_log.vi"("Header message"=w419) -> ()
            n191 = Not(x="stop") -> (.not. x?=w422:bool)
          }
          frame #22 {
            n192 = call "Update_Ch_Discription_server.vi"("Mode"=T7."Read Global then Clear") -> ("Channels to update Out"=w425:T8[])  [unwired: 2 in]
            n193 = Array Size(array=w425) -> (size(s)=w427:i32)
            n194 = Equal To 0?(x=w427) -> (x = 0?=w426:bool)
            n195 = case shown="False" w426 {
              tunnel: w424 -> [w432 _]
              tunnel: w425 -> [w431 _]
              frame False {
                n196 = global read "Channel_Description_Global.vi" "Channel Description"() -> (w430:T8[])
                n197 = for {
                  tunnel: w432 -> [w439]
                  tunnel: w431 -> [w436] mode=indexing
                  shift-right: [w435] -> w429
                  shift-left: w430 -> [w438]
                  n198 = Unbundle By Name(w436) -> ("Ch Name"=w437:string)
                  n199 = Search 1D Array(1D array=w439, element=w437) -> (index of element=w433:i32)  [unwired: 1 out]
                  n200 = Less Than 0?(x=w433) -> (x < 0?=w434:bool)
                  n201 = case shown="False" w434 {
                    tunnel: w438 -> [w443 w446]
                    tunnel: w436 -> [w442 w444]
                    tunnel: [w441 w445] -> w435
                    tunnel: w433 -> [w440 _]
                    frame False {
                      n202 = Replace Array Subset(array=w443, new element=w442, index=w440) -> (w441:T8[])
                    }
                    frame True {
                      n203 = Build Array (concatenate)(w446, w444) -> (w445:T8[])
                    }
                  }
                }
                n204 = global write "Channel_Description_Global.vi" "Channel Description"(w429) -> ()
              }
              frame True {
              }
            }
          }
          frame #23 {
            n205 = case shown="True" "Load setup from file" {
              frame False {
              }
              frame True {
                n206 = local write "Save Current setup"(TRUE ("Save Current setup")) -> ()
                n207 = call "Read_Write_ADAM_setup.vi"("Mode"=T1."Load ADAM setup from excel file") -> ()  [unwired: 4 out]
              }
            }
          }
          frame #24 {
            n208 = case shown="0" w452 {
              tunnel: w451 -> [_ _]
              frame 0 {
                n209 = global read "Constants_global.vi" "EnFlo SW Folder"() -> (w457:path)
                n210 = Build Path(base path=w457, name or relative path=path "ADAM Client/ADAM client VIs/Plot_Server_Data.vi") -> (appended path=w454:path)
                n211 = call "Load_Comparitor_Cluster.vi"() -> ()  [unwired: 12 in]
                n212 = Build Path(base path=w457, name or relative path=path "ADAM Server/Log_ADAM_scan_table.vi") -> (appended path=w455:path)
                n213 = Build Array(w455, w454) -> (w453:path[])
                n214 = for {
                  tunnel: w453 -> [w459] mode=indexing
                  n215 = Open VI Reference(vi path=w459) -> (vi reference=w463:refnum<vi>, error out=w462:errorcluster)  [unwired: 2 in, 3 out]
                  n216 = property class="VI"(reference=w463, error in=w462, "Front Panel Window:Open"=TRUE) -> (reference out=w460:refnum<vi>, error out=w461:errorcluster)
                  n217 = invoke class="VI" method="Run VI"(reference=w460, error in=w461, "Wait until done"=FALSE) -> (reference out=w467:refnum<vi>, error out=w466:errorcluster)  [unwired: 2 in, 3 out]
                  n218 = Close Reference(reference=w467, error in (no error)=w466) -> ()  [unwired: 1 out]
                }
              }
              frame 1, Default {
              }
            }
          }
        }
        "History length" <- w53
      }
    }
    frame #5 {
      w468 = FALSE  # Set Watchdogs
      n219 = call "Set_Adam_Watchdogs.vi"("Set Watchdogs"=w468) -> ()  [unwired: 1 out]
      n220 = call "Read_Write_ADAM_setup.vi"("Mode"=T1."Save ADAM setup to excel file") -> ()  [unwired: 4 out]
    }
  }
